vi "add_remove_change.vi"() -> ()   [LabVIEW 2015]
uses:
  ComponentType.ctl
panel:
  out "Action":enum16{"Add", "Remove", "Swap"}(ring)
  in  "Component Type":T1
  in  "New Components":string[](array[string])
  in  "Old Components":string[](array[string])
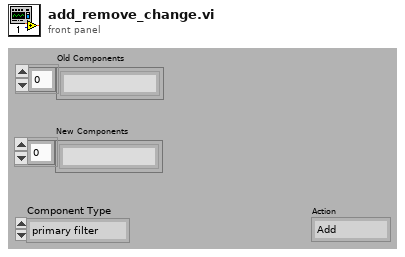
[diagram p1: front panel]
types:
  T1 = typedef "ComponentType.ctl" = enum16{"primary filter", "secondary filter", "grating", "slit/mask"}
  T2 = cluster{"Component Type":T1, "Action":enum16{"Add", "Remove", "Swap"}, "Position":i32}[]
  T3 = cluster{"Component Type":T1, "Action":enum16{"Add", "Remove", "Swap"}, "Position":i32}
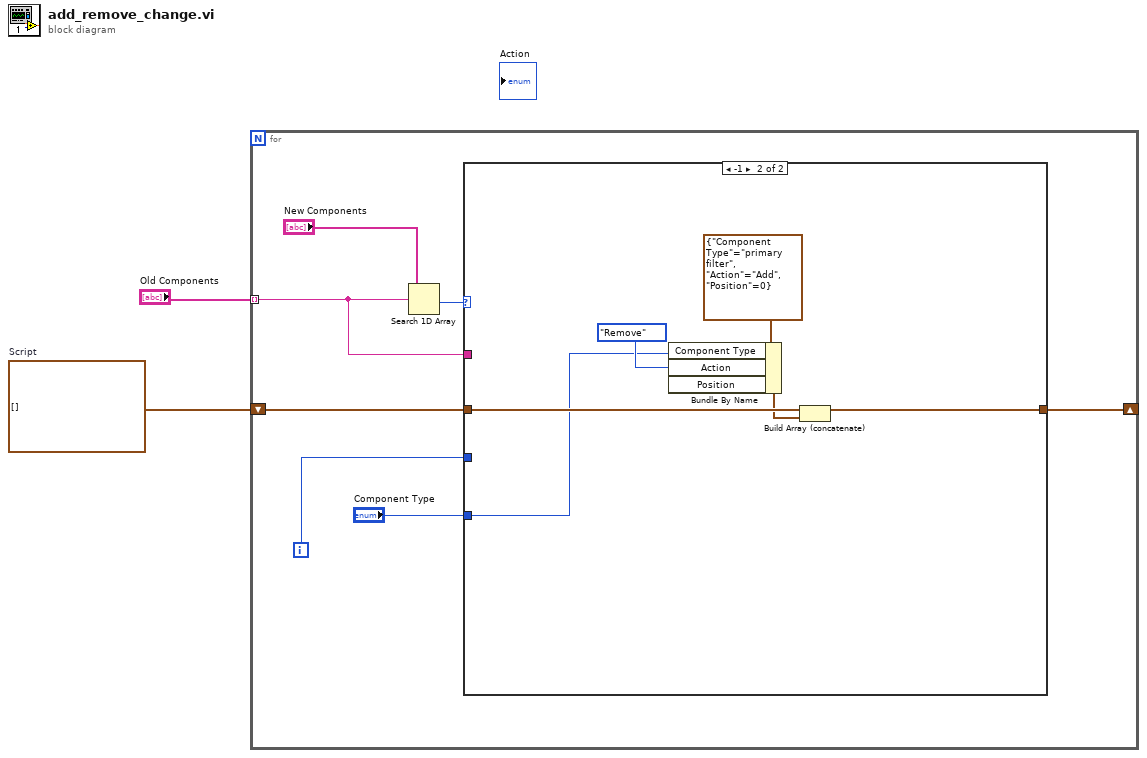
[diagram p0: block diagram]
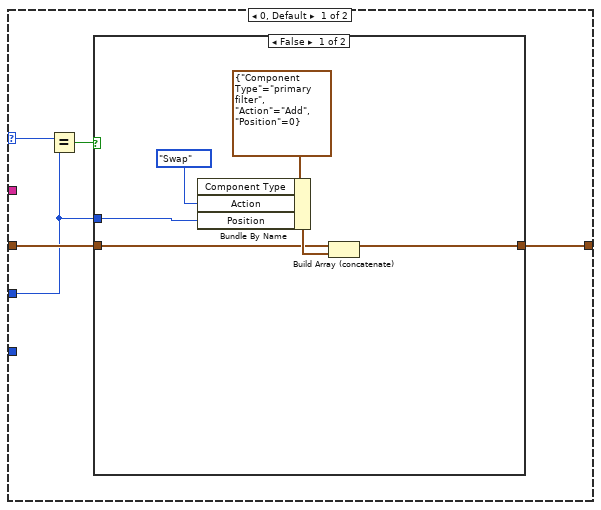
[diagram p2: hidden frame]
diagram:
  w2 = T2 []  # Script
  n1 = for {
    tunnel: "Old Components" -> [w7] mode=indexing
    shift-right: [w4] -> _
    shift-left: w2 -> [w8]
    i -> [w6]
    n2 = Search 1D Array(1D array="New Components", element=w7) -> (index of element=w9:i32)  [unwired: 1 in]
    n3 = case shown="-1" w9 {
      selector: w9 -> [w14 _]
      tunnel: w8 -> [w12 w27]
      tunnel: w7 -> [_ _]
      tunnel: w6 -> [w10 _]
      tunnel: [w11 w26] -> w4
      tunnel: "Component Type" -> [_ w22]
      frame 0, Default {
        n4 = Equal?(x=w14, y=w10) -> (x = y?=w13:bool)
        n5 = case shown="False" w13 {
          tunnel: w12 -> [w17 w21]
          tunnel: [w16 w21] -> w11
          tunnel: w10 -> [w15 _]
          frame False {
            n6 = Bundle By Name(cluster=T3 {"Component Type"=enum."primary filter", "Action"=enum."Add", "Position"=0}, "Action"=enum16{"Add", "Remove", "Swap"}."Swap", "Position"=w15) -> (w19:T3)  [unwired: 1 in]
            n7 = Build Array (concatenate)(w17, w19) -> (w16:T2)
          }
          frame True {
          }
        }
      }
      frame -1 {
        n8 = Bundle By Name(cluster=T3 {"Component Type"=enum."primary filter", "Action"=enum."Add", "Position"=0}, "Component Type"=w22, "Action"=enum16{"Add", "Remove", "Swap"}."Remove") -> (w24:T3)  [unwired: 1 in]
        n9 = Build Array (concatenate)(w27, w24) -> (w26:T2)
      }
    }
  }
